vi "_TablePage.vi"(11 "DB Ref":T2) -> (2 "Value String":string, 3 "Boolean":bool)   [LabVIEW 2017]
uses:
  TagDB/Typedef/TagDB.ctl
  d04a7fc7-71e9-4228-902b-2c8062d38224.vi
  TagDB/_Support/DataAccess/_NameCacher.vi
  TagDB/_Support/DataAccess/TagDB Ref to DVR.vi
  TagDB/_Support/Error/_[error50000]Invalid DB REF.vi
  TagDB/_Support/Change Detector/TagDB dbChanged.vi
  TagDB/_Support/URL/TRIM-BOTH-SPACE.vi
  TagDB/_Support/Error/_[error50002]Invalid DataType.vi
  TagDB/TagDB.lvlib
panel:
  out "Valid?":bool
  out "Name":string
  out "DataItemFlag":timestamp
  out "DataChangeFlag":timestamp
  out "Array":T1(array[cluster])
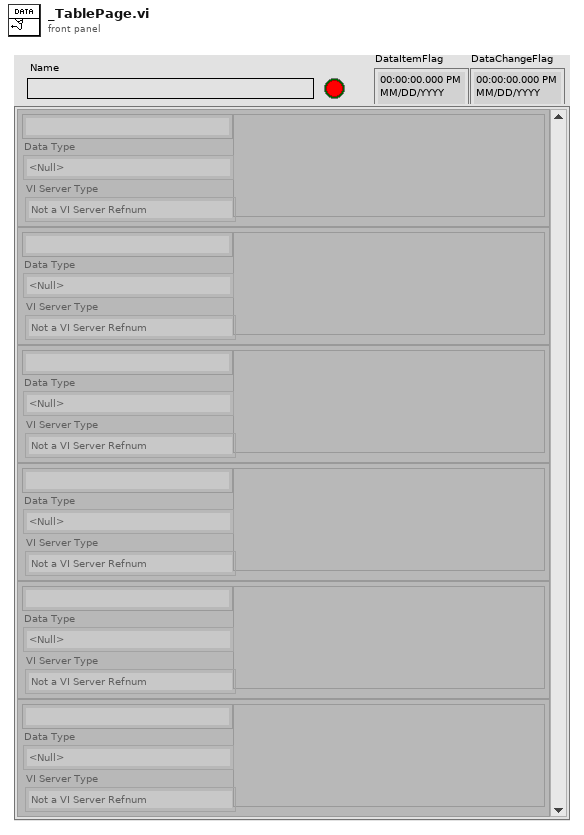
[diagram p1: front panel]
types:
  T1 = cluster{"Tag":string, "Data Type":enum8{"<Null>", "I8", "I16", "I32", "I64", "U8", "U16", "U32", "U64", "SGL", "DBL", "EXT", "CSG", "CDB", "CXT", "0x0F", "0x10", "0x11", "0x12", "0x13", "0x14", "Enum U8", "Enum U16", "Enum U32", "Enum U64", "SGL PQ", "DBL PQ", "EXT PQ", "CSG PQ", "CDB PQ", "CXT PQ", "0x1F", "0x20", "Boolean", "0x22", "0x23", "0x24", "0x25", "0x26", "0x27", "0x28", "0x29", "0x2A", "0x2B", "0x2C", "0x2D", "0x2E", "0x2F", "String", "0x31", "Path", "Pict", "0x34", "0x35", "0x36", "DAQ", "0x38", "0x39", "0x3A", "0x3B", "0x3C", "0x3D", "0x3E", "0x3F", "Array", "0x41", "0x42", "0x43", "0x44", "0x45", "0x46", "0x47", "0x48", "0x49", "0x4A", "0x4B", "0x4C", "0x4D", "0x4E", "0x4F", "Cluster", "0x51", "0x52", "Variant", "Waveform", "0x55", "0x56", "0x57", "0x58", "0x59", "0x5A", "0x5B", "0x5C", "0x5D", "0x5E", "0x5F", "0x60", "0x61", "0x62", "0x63", "0x64", "0x65", "0x66", "0x67", "0x68", "0x69", "0x6A", "0x6B", "0x6C", "0x6D", "0x6E", "0x6F", "Refnum"}, "VI Server Type":enum16{"Not a VI Server Refnum", "Control", "VI", "Application", "Splitter", "Pane"}, "Value":variant}[]
  T2 = typedef "TagDB.lvlib/TagDB.ctl" = refnum<k1>
  T3 = cluster{"Reference":refnum<vi>, "ClassName":string, "Value":variant}
  T4 = enum8{"<Null>", "I8", "I16", "I32", "I64", "U8", "U16", "U32", "U64", "SGL", "DBL", "EXT", "CSG", "CDB", "CXT", "0x0F", "0x10", "0x11", "0x12", "0x13", "0x14", "Enum U8", "Enum U16", "Enum U32", "Enum U64", "SGL PQ", "DBL PQ", "EXT PQ", "CSG PQ", "CDB PQ", "CXT PQ", "0x1F", "0x20", "Boolean", "0x22", "0x23", "0x24", "0x25", "0x26", "0x27", "0x28", "0x29", "0x2A", "0x2B", "0x2C", "0x2D", "0x2E", "0x2F", "String", "0x31", "Path", "Pict", "0x34", "0x35", "0x36", "DAQ", "0x38", "0x39", "0x3A", "0x3B", "0x3C", "0x3D", "0x3E", "0x3F", "Array", "0x41", "0x42", "0x43", "0x44", "0x45", "0x46", "0x47", "0x48", "0x49", "0x4A", "0x4B", "0x4C", "0x4D", "0x4E", "0x4F", "Cluster", "0x51", "0x52", "Variant", "Waveform", "0x55", "0x56", "0x57", "0x58", "0x59", "0x5A", "0x5B", "0x5C", "0x5D", "0x5E", "0x5F", "0x60", "0x61", "0x62", "0x63", "0x64", "0x65", "0x66", "0x67", "0x68", "0x69", "0x6A", "0x6B", "0x6C", "0x6D", "0x6E", "0x6F", "Refnum"}
  T5 = enum16{"Not a VI Server Refnum", "Control", "VI", "Application", "Splitter", "Pane"}
  T6 = cluster{string, "type":enum8{"<Null>", "I8", "I16", "I32", "I64", "U8", "U16", "U32", "U64", "SGL", "DBL", "EXT", "CSG", "CDB", "CXT", "0x0F", "0x10", "0x11", "0x12", "0x13", "0x14", "Enum U8", "Enum U16", "Enum U32", "Enum U64", "SGL PQ", "DBL PQ", "EXT PQ", "CSG PQ", "CDB PQ", "CXT PQ", "0x1F", "0x20", "Boolean", "0x22", "0x23", "0x24", "0x25", "0x26", "0x27", "0x28", "0x29", "0x2A", "0x2B", "0x2C", "0x2D", "0x2E", "0x2F", "String", "0x31", "Path", "Pict", "0x34", "0x35", "0x36", "DAQ", "0x38", "0x39", "0x3A", "0x3B", "0x3C", "0x3D", "0x3E", "0x3F", "Array", "0x41", "0x42", "0x43", "0x44", "0x45", "0x46", "0x47", "0x48", "0x49", "0x4A", "0x4B", "0x4C", "0x4D", "0x4E", "0x4F", "Cluster", "0x51", "0x52", "Variant", "Waveform", "0x55", "0x56", "0x57", "0x58", "0x59", "0x5A", "0x5B", "0x5C", "0x5D", "0x5E", "0x5F", "0x60", "0x61", "0x62", "0x63", "0x64", "0x65", "0x66", "0x67", "0x68", "0x69", "0x6A", "0x6B", "0x6C", "0x6D", "0x6E", "0x6F", "Refnum"}, "Enum":enum16{"Not a VI Server Refnum", "Control", "VI", "Application", "Splitter", "Pane"}, "Variant":variant}
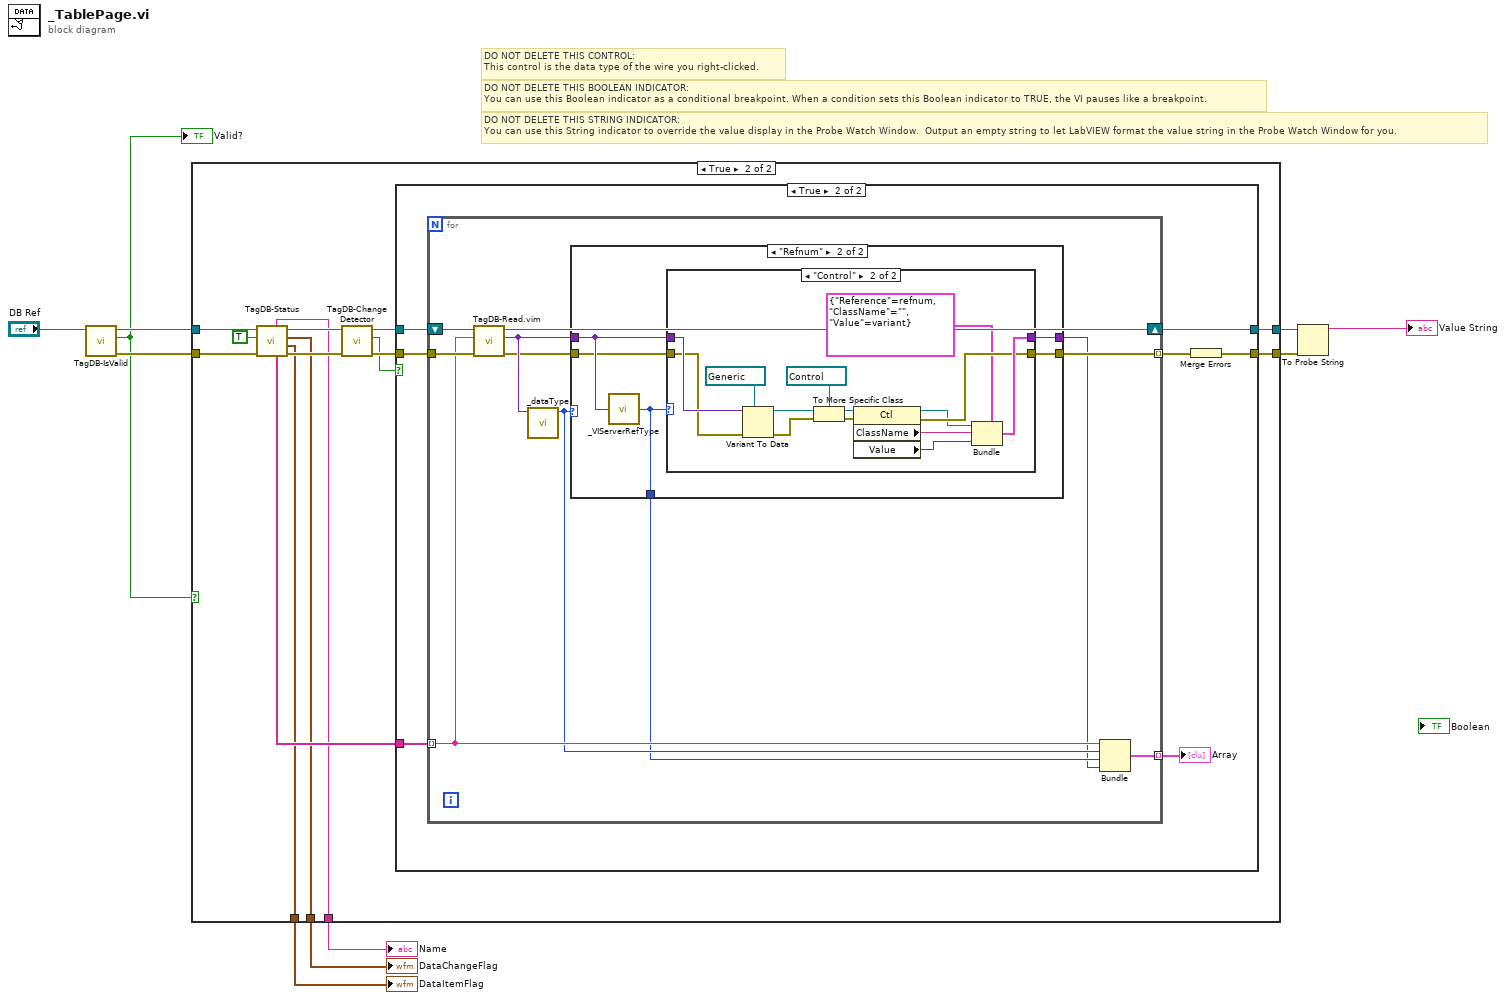
[diagram p0: block diagram]
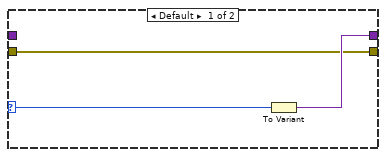
[diagram p5: hidden frame]
diagram:
  # "DO NOT DELETE THIS STRING INDICATOR: \nYou can use this String indicator to override the value display in the Probe Watch Window.  Output an empty string to let LabVIEW format the value string in the Probe Watch Window for you."
  # "DO NOT DELETE THIS BOOLEAN INDICATOR: \nYou can use this Boolean indicator as a conditional breakpoint. When a condition sets this Boolean indicator to TRUE, the VI pauses like a breakpoint."
  # "DO NOT DELETE THIS CONTROL: \nThis control is the data type of the wire you right-clicked."
  n1 = call "TagDB-IsValid.vi"("TagDB"="DB Ref") -> ("error out"=w7:errorcluster, "valid TagDB?"=w4:bool, "TagDB(dup)"=w8:T2)  [unwired: 8 in]
  "Valid?" <- w4
  n2 = case shown="True" w4 {
    tunnel: w8 -> [w12 w21]
    tunnel: w7 -> [w11 w19]
    tunnel: [w12 w26] -> w6
    tunnel: [w11 w25] -> w5
    tunnel: [_ w15] -> w3
    tunnel: [_ w13] -> w2
    tunnel: [_ w14] -> w1
    frame False {
    }
    frame True {
      n3 = call "TagDB-Status.vi"("error in (no error)"=w19, "return elements? (F)"=TRUE, "DB Ref"=w21) -> ("error out"=w17:errorcluster, "Item Change Timestamp"=w15:timestamp, "Global Change Timestamp"=w14:timestamp, "DB Ref(dup)"=w20:T2, "DB items"=w16:string[], "db name"=w13:string)  [unwired: 3 in]
      n4 = call-poly "TagDB-Change Detector.vi"("error in (no error)"=w17, "DB Ref"=w20) -> ("error in (no error) (dup)"=w23:errorcluster, "changed?"=w22:bool, "DB Ref (dup)"=w24:T2)  [unwired: 7 in]
      n5 = case shown="True" w22 {
        tunnel: [w28 w35] -> w26
        tunnel: [w27 w29] -> w25
        tunnel: w16 -> [_ w33]
        tunnel: w24 -> [w28 w32]
        tunnel: w23 -> [w27 w31]
        frame False {
        }
        frame True {
          n6 = for {
            tunnel: w33 -> [w41] mode=indexing
            shift-right: [w46] -> w35
            shift-left: w32 -> [w36]
            tunnel: [w37] -> w30 mode=indexing
            tunnel: w31 -> [w44]
            tunnel: [w45] -> w34 mode=indexing
            n7 = call "TagDB-Read.vim"("error in (no error)"=w44, "name"=w41, "TagDB"=w36) -> ("error out"=w42:errorcluster, "Value"=w43:variant, "TagDB(dup)"=w46:T2)  [unwired: 3 in, 3 out]
            n8 = call "_dataType.vi"("Type"=w43) -> ("type"=w40:T4)  [unwired: 10 in]
            n9 = case shown="\"Refnum\"" w40 {
              tunnel: [w48 w53] -> w38
              tunnel: w43 -> [w48 w52]
              tunnel: w42 -> [w47 w51]
              tunnel: [w47 w50] -> w45
              tunnel: [_ w49] -> w39
              frame Default {
              }
              frame "Refnum" {
                n10 = call "_VIServerRefType.vi"("Data"=w52) -> ("Enum"=w49:T5)  [unwired: 4 in]
                n11 = case shown="\"Control\"" w49 {
                  selector: w49 -> [w56 _]
                  tunnel: [w55 w61] -> w53
                  tunnel: w52 -> [_ w70]
                  tunnel: w51 -> [w54 w60]
                  tunnel: [w54 w59] -> w50
                  frame Default {
                    n12 = To Variant(anything=w56) -> (Variant=w55:variant)
                  }
                  frame "Control" {
                    n13 = Variant To Data(error in=w60, type=refnum<vi> refnum ("value"), Variant=w70) -> (data=w68:refnum<vi>, error out=w67:errorcluster)
                    n14 = To More Specific Class(target class=refnum<vi> refnum ("value"), reference=w68, error in=w67) -> (specific class reference=w65:refnum<vi>, error out=w64:errorcluster)
                    n15 = property class="Ctl"(reference=w65, error in=w64) -> (reference out=w58:refnum<vi>, error out=w59:errorcluster, "ClassName"=w63:string, "Value"=w62:variant)
                    n16 = Bundle(cluster=T3 {"Reference"=refnum, "ClassName"="", "Value"=variant}, "Reference"=w58, "ClassName"=w63, "Value"=w62) -> (w61:T3)
                  }
                }
              }
            }
            n17 = Bundle(w41, "type"=w40, "Enum"=w39, "Variant"=w38) -> (w37:T6)  [unwired: 1 in]
          }
          "Array" <- w30
          n18 = Merge Errors(w34) -> (w29:errorcluster)
        }
      }
    }
  }
  "DataChangeFlag" <- w1
  "DataItemFlag" <- w3
  "Name" <- w2
  n19 = To Probe String(4:w5, 7:w6) -> (3:→"Value String":string)  [unwired: 1 in, 1 out]
